vi "Autoselect_Drivers.vi"(8 "error in (no error)":errorcluster, 11 "IB_MSI in":refnum<class "IB_MSI.lvclass">) -> (0 "error out":errorcluster, 2 "autoSelect?":bool, 3 "IB_MSI out":refnum<class "IB_MSI.lvclass">)   [LabVIEW 2020, in "IB_MSI.lvclass"]
uses:
  <vilib>/AppBuilder/IB_Classes/MSI/IB_MSI.lvclass
  <vilib>/AppBuilder/IB_Classes/MSI/IB_MSI.lvclass/IB_MSI.ctl
  <vilib>/AppBuilder/IB_Classes/DistPart/IB_DistPart.lvclass
  <vilib>/AppBuilder/IB_Classes/Installer/Installer.lvclass
  <vilib>/AppBuilder/IB_Classes/Source/Container/Build/IB_Source_Build.lvclass
  <vilib>/Utility/lvfile.llb/LVFileType.ctl
  <vilib>/Utility/lvfile.llb/NI_FileType.lvlib
  <resource>/Framework/Providers/Builds/Installer/CDK_sTypeDef_FindProduct.ctl
  <vilib>/AppBuilder/AB_Dependency.ctl
  <vilib>/AppBuilder/IB_Classes/Source/IB_Source.lvclass
  e:/builds/penguin/labview/branches/2020/dev/dist/vi.lib/AppBuilder/IB_Classes/Installer/Installer.lvclass
  e:/builds/penguin/labview/branches/2020/dev/dist/vi.lib/AppBuilder/IB_Classes/MSI/IB_MSI.lvclass
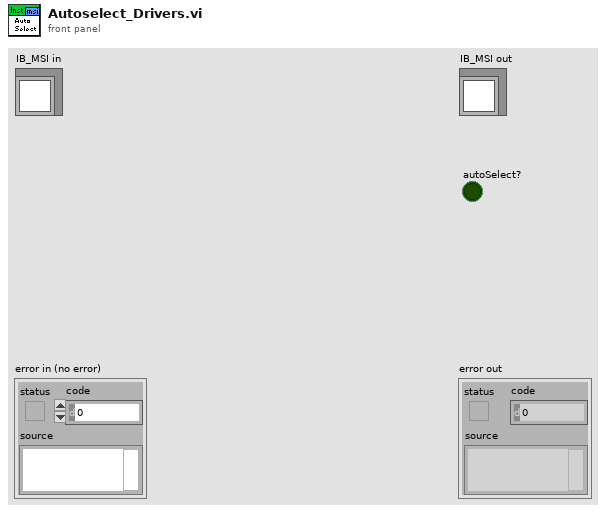
[diagram p1: front panel]
types:
  T1 = typedef "CDK_sTypeDef_FindProduct.ctl" = enum16{"LabVIEW RTE", "DataSocket", "USI", "CVI RTE", "LVDeployableLic"}
  T2 = typedef "AB_Dependency.ctl" = cluster{"path":path, "delimited name":string, "type":T3}
  T3 = typedef "NI_FileType.lvlib/LVFileType.ctl" = enum32{"Invalid file", "Unknown type", "Instrument", "Control", "Polymorphic VI", "Project", "Library", "LVClass", "XControl", "XNode", "Shared library", ".NET assembly", "ActiveX interface", "CIN", "Run-time menu", "Palette menu", "Help file", "LLB", "XNode Edit Dependency", "Class Private Data Control", "Statechart", "MathScript .m file", "Ladder Diagram", "LVLibp", "XNode Build Dependency"}
  T4 = typedef "IB_Installer.ctl" = cluster{"Destination":refnum<class "IB_Destination.lvclass">[], "Source":refnum<class "IB_Source.lvclass">[], "buildObject":T5, "defaultDir":string, "platform":string, "author":string, "productName":string, "buildSpecName":string, "hide":bool, "requireLVDevSys":bool, "autoIncrement":bool, "includeError":bool, "readmeID":string, "buildLocation":path, "readmePath":path, "mediaSize":u16, "language":T6, "productVersion":T7, "preview":bool, "programmatic":bool, "progressBarEvents":T8, "userLog_Path":path, "shortcutAddresses":T10[], "EXE_Install Address":string, "EXE_Uninstall Address":string, "additional NIPaths":refnum<class "Dest_NI_NIPath.lvclass">[], "web service itemIDs":string[], "installerName":string}
  T5 = typedef "ItemRef.ctl" = u64
  T6 = typedef "CDK_sTypeDef_Languages.ctl" = u16
  T7 = typedef "CDK_sTypeDef_ProductVersion.ctl" = cluster{"Major":u8, "Minor":u8, "Update":u16}
  T8 = typedef "provcom_ProgressBar_Events.ctl" = cluster{"newJob":refnum<user-event>, "newItem":refnum<user-event>, "errorMsg":T9, "cancel":refnum<user-event>}
  T9 = typedef "mxLvBuildError.ctl" = refnum<user-event>
  T10 = typedef "CDK_sTypeDef_ShortcutAddress.ctl" = cluster{"file":string, "shortcut":string}
  T11 = typedef "IB_Source.ctl" = cluster{"name":string, "sourceTag":string, "destTag":string, "path":path, "eng_installPath":string, "UI_inBuild?":bool, "str ref?":bool}
  T12 = typedef "IB_DistPart.ctl" = cluster{"ProductName":string, "ProductId":string, "ProductDescription":string, "Path":path, "FlavorId":string, "DistTitle":string, "UpgradeCode":string, "Flavors":T13[], "SoftDependencies":refnum<class "IB_SoftDependency.lvclass">[], "DistPartType":T14}
  T13 = typedef "IB_FlavorInfo.ctl" = cluster{"FlavorId":string, "Visible?":bool, "Name":string, "Descrp":string, "Cost(MB)":i32, "hasLicMgmt?":bool, "DistPartType":T14}
  T14 = typedef "IB_DistPartType.ctl" = enum16{"Full", "Runtime"}
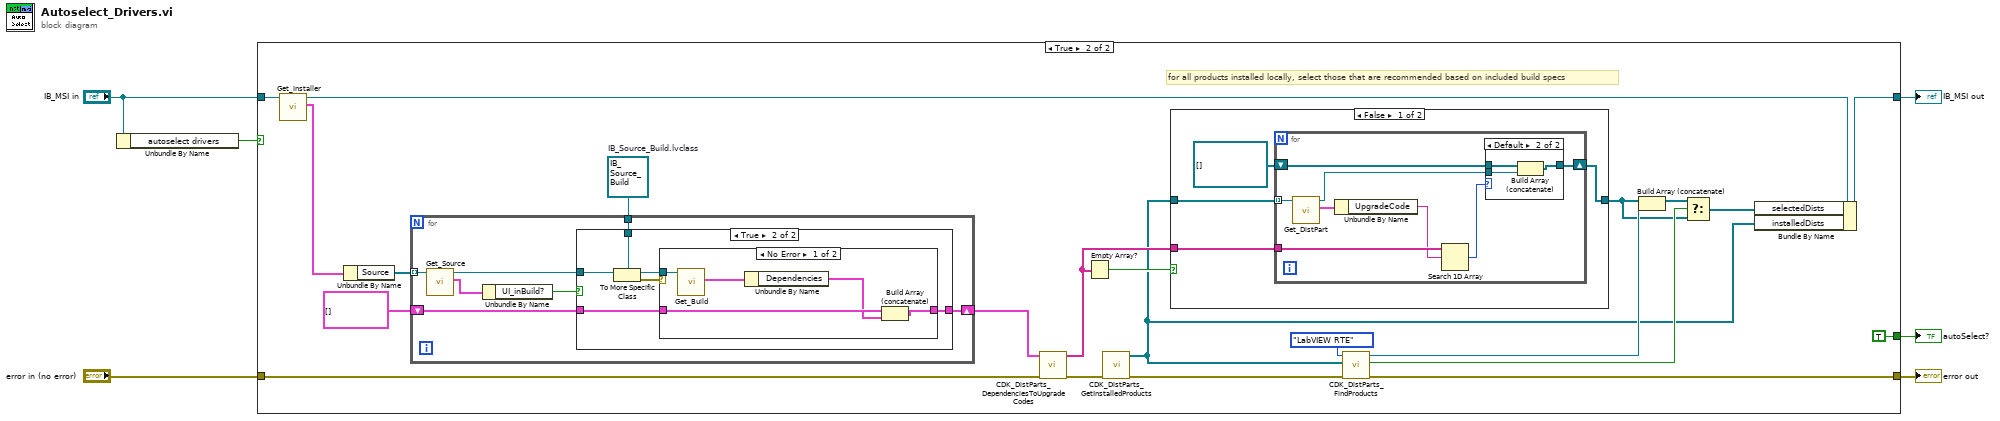
[diagram p0: block diagram]
diagram:
  n1 = Unbundle By Name("IB_MSI in") -> ("autoselect drivers"=w2:bool)
  n2 = case shown="True" w2 {
    tunnel: [w8 w20] -> w6
    tunnel: "error in (no error)" -> [w7 w30]
    tunnel: [w7 w29] -> w4
    tunnel: "IB_MSI in" -> [w8 w28]
    tunnel: [_ TRUE] -> w1
    frame False {
    }
    frame True {
      w24 = refnum<class "IB_Source_Build.lvclass"> refnum  # IB_Source_Build.lvclass
      # "for all products installed locally, select those that are recommended based on included build specs"
      n3 = call <vilib>:"Get_Installer.vi"("Installer in"=w28) -> ("data"=w26:T4, "Installer out"=w27:refnum<class "IB_MSI.lvclass">)  [unwired: 8 in, 1 out]
      n4 = Unbundle By Name(w26) -> ("Source"=w25:refnum<class "IB_Source.lvclass">[])
      n5 = for {
        tunnel: w25 -> [w50] mode=indexing
        tunnel: w24 -> [w53]
        shift-right: [w51] -> w23
        shift-left: T2[] [] ("Dependencies") -> [w52]
        n6 = call <vilib>:"Get_Source.vi"("IB_Source in"=w50) -> ("data"=w48:T11, "IB_Source out"=w49:refnum<class "IB_Source.lvclass">)  [unwired: 8 in, 1 out]
        n7 = Unbundle By Name(w48) -> ("UI_inBuild?"=w47:bool)
        n8 = case shown="True" w47 {
          tunnel: w53 -> [_ w60]
          tunnel: w52 -> [w54 w58]
          tunnel: [w54 w57] -> w51
          tunnel: w49 -> [_ w55]
          frame False {
          }
          frame True {
            n9 = To More Specific Class(target class=w60, reference=w55) -> (specific class reference=w59:refnum<class "IB_Source_Build.lvclass">, error out=w56:errorcluster)  [unwired: 1 in]
            n10 = case shown="No Error" w56 {
              tunnel: w59 -> [w65 _]
              tunnel: w58 -> [w64 w66]
              tunnel: [w63 w66] -> w57
              frame No Error {
                n11 = call <vilib>:"Get_Build.vi"("IB_Source_Build in"=w65) -> ("data"=w62:cluster{"Dependencies":T2[]})  [unwired: 8 in, 2 out]
                n12 = Unbundle By Name(w62) -> ("Dependencies"=w61:T2[])
                n13 = Build Array (concatenate)(w64, w61) -> (w63:T2[])
              }
              frame Error {
              }
            }
          }
        }
      }
      n14 = call <vilib>:"CDK_DistParts_DependenciesToUpgradeCodes.vi"("error in (no error)"=w30, "calculated dependencies"=w23) -> ("error out"=w9:errorcluster, "upgrade codes"=w19:string[])  [unwired: 8 in]
      n15 = Empty Array?(array=w19) -> (empty?=w18:bool)
      n16 = call <resource>:"CDK_DistParts_GetInstalledProducts.vi"("ErrIn"=w9) -> ("ErrOut"=w10:errorcluster, "installed products"=w11:refnum<class "IB_DistPart.lvclass">[])  [unwired: 9 in]
      n17 = case shown="False" w18 {
        tunnel: w19 -> [w34 _]
        tunnel: [w31 _] -> w12
        tunnel: w11 -> [w33 _]
        frame False {
          n18 = for {
            tunnel: w33 -> [w42] mode=indexing
            tunnel: w34 -> [w40]
            shift-right: [w36] -> w31
            shift-left: refnum<class "IB_DistPart.lvclass">[] [] ("installed products") -> [w37]
            n19 = call <vilib>:"Get_DistPart.vi"("Class in"=w42) -> ("data"=w41:T12, "Class out"=w35:refnum<class "IB_DistPart.lvclass">)  [unwired: 8 in, 1 out]
            n20 = Unbundle By Name(w41) -> ("UpgradeCode"=w39:string)
            n21 = Search 1D Array(1D array=w40, element=w39) -> (index of element=w38:i32)  [unwired: 1 in]
            n22 = case shown="Default" w38 {
              tunnel: [w43 w45] -> w36
              tunnel: w37 -> [w43 w46]
              tunnel: w35 -> [_ w44]
              frame -1 {
              }
              frame Default {
                n23 = Build Array (concatenate)(w46, w44) -> (w45:refnum<class "IB_DistPart.lvclass">[])
              }
            }
          }
        }
        frame True {
        }
      }
      n24 = call <resource>:"CDK_DistParts_FindProducts.vi"("ErrIn"=w10, "InstalledProducts"=w11, "ProductName"=CDK_sTypeDef_FindProduct."LabVIEW RTE") -> ("ErrOut"=w29:errorcluster, "Found?"=w14:bool, "RunTime Engine"=w15:refnum<class "IB_DistPart.lvclass">)  [unwired: 5 in, 1 out]
      n25 = Build Array (concatenate)(w12, w15) -> (w13:refnum<class "IB_DistPart.lvclass">[])
      n26 = Select(t=w13, s=w14, f=w12) -> (s? t:f=w16:refnum<class "IB_DistPart.lvclass">[])
      n27 = Bundle By Name(cluster=w27, "selectedDists"=w16, "installedDists"=w11) -> (w20:refnum<class "IB_MSI.lvclass">)
    }
  }
  "error out" <- w4
  "IB_MSI out" <- w6
  "autoSelect?" <- w1
